vi "config_burst.vi"(0 "VISA resource name":refnum<visa-resource-name>="TRIG", 1 "burst count":i32, 2 "burst period (s)":dbl, 3 "error in (no error)":errorcluster, 4 "Burst enable?":bool) -> (5 "VISA resource name out":refnum<visa-resource-name>, 7 "error out":errorcluster)   [LabVIEW 2011]
doc: "Sets he burst period and the burst count. \n\nSets he burst count. When burst mode is enabled, the DG645 \noutputs burst count delay cycles per trigger.\n\nThe burst period sets the time between delay cycles during a burst. \nThe burst period may range from 100 ns to 2000 – 10 ns in 10 ns steps."
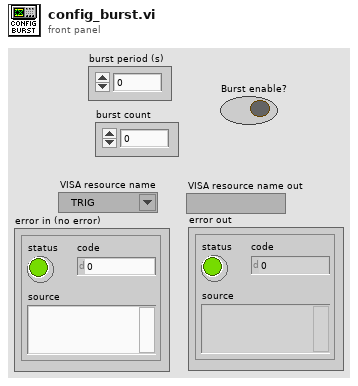
[diagram p1: front panel]
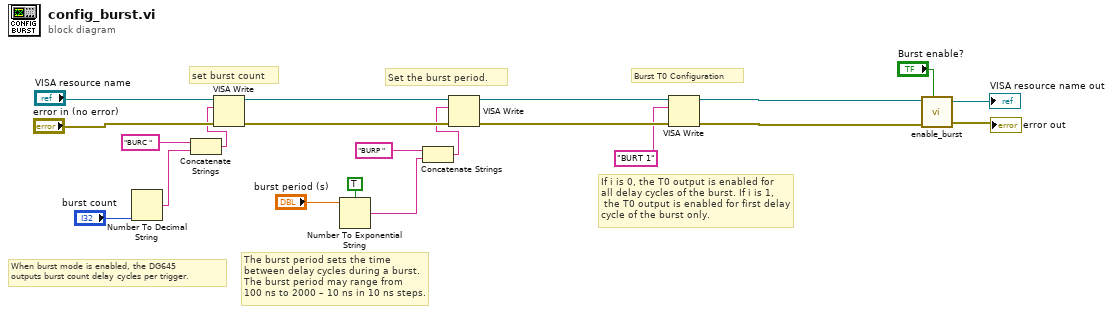
[diagram p0: block diagram]
diagram:
  # "If i is 0, the T0 output is enabled for \nall delay cycles of the burst. If i is 1,\n the T0 output is enabled for first delay \ncycle of the burst only."
  # "Burst T0 Configuration"
  # "Set the burst period."
  # "When burst mode is enabled, the DG645 \noutputs burst count delay cycles per trigger."
  # "The burst period sets the time \nbetween delay cycles during a burst. \nThe burst period may range from \n100 ns to 2000 – 10 ns in 10 ns steps."
  # "set burst count"
  n1 = Number To Decimal String(number="burst count") -> (decimal integer string=w13:string)  [unwired: 1 in]
  n2 = Concatenate Strings("BURC " ("Query 2"), w13) -> (w17:string)
  n3 = VISA Write(VISA resource name="VISA resource name", write buffer=w17, error in (no error)="error in (no error)") -> (VISA resource name out=w15:refnum<visa-resource-name>, error out=w18:errorcluster)  [unwired: 1 out]
  n4 = Number To Exponential String(number="burst period (s)", 1:TRUE ("use system decimal point (T)")) -> (E-format string=w11:string)  [unwired: 2 in]
  n5 = Concatenate Strings("BURP " ("Query 2"), w11) -> (w14:string)
  n6 = VISA Write(VISA resource name=w15, write buffer=w14, error in (no error)=w18) -> (VISA resource name out=w3:refnum<visa-resource-name>, error out=w7:errorcluster)  [unwired: 1 out]
  n7 = VISA Write(VISA resource name=w3, write buffer="BURT 1", error in (no error)=w7) -> (VISA resource name out=w2:refnum<visa-resource-name>, error out=w4:errorcluster)  [unwired: 1 out]
  n8 = call "enable_burst.vi"("VISA resource name"=w2, "error in (no error)"=w4, "Burst enable?"="Burst enable?") -> ("VISA resource name out"=→"VISA resource name out":refnum<visa-resource-name>, "error out"=→"error out":errorcluster)  [unwired: 3 in]
